vi "LDF Parser File.vi"(7 "pLDFFileName":string, 9 "isMaster":u8, 10 "LINIndex":i32, 11 "DevHandle":i32) -> (3 "function return":u64, 5 "pLDFFileName out":string)   [LabVIEW 2010, in "ldf_parser.lvlib"]
doc: "long long WINAPI LDF_ParserFile(int DevHandle, int LINIndex, unsigned char isMaster, char* pLDFFileName);"
uses:
  ldf_parser.lvlib
  USB2XXX/trunk/USB2XXX/USB2XXX/vs2019/Release/USB2XXX.dll
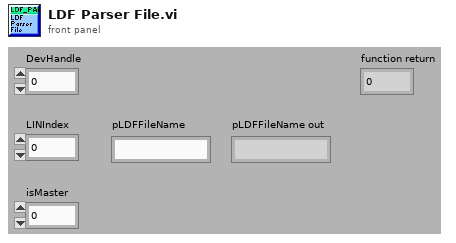
[diagram p1: front panel]
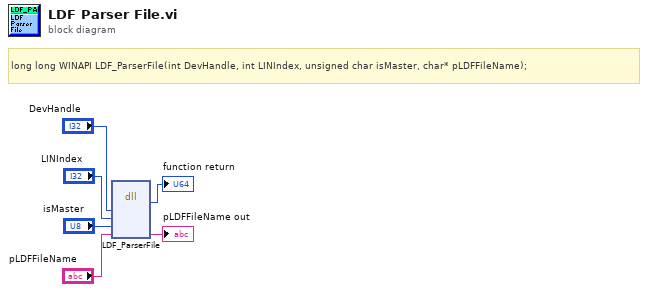
[diagram p0: block diagram]
diagram:
  # "long long WINAPI LDF_ParserFile(int DevHandle, int LINIndex, unsigned char isMaster, char* pLDFFileName);"
  n1 = dll-call lib="E:/Projects/USB2XXX/trunk/USB2XXX/USB2XXX/vs2019/Release/USB2XXX.*" fn="LDF_ParserFile"("DevHandle"="DevHandle", "LINIndex"="LINIndex", "isMaster"="isMaster", "pLDFFileName"="pLDFFileName") -> (→"function return":u64, "pLDFFileName"=→"pLDFFileName out":string)  [unwired: 6 in, 2 out]
